vi "Calculate_10Minutes_Averages.vi"(0 "Current time":dbl) -> ()   [LabVIEW 2013]
uses:
  <vilib>/Analysis/baseanly.llb/Mean (DBL).vi
  Globals/Weather_Queues.vi
  <vilib>/Analysis/NI_AALBase.lvlib
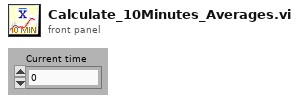
[diagram p1: front panel]
types:
  T1 = cluster{"Weather data (5s)":refnum<queue>, "Database queue":refnum<queue>, "Message queue":refnum<queue>, "Settings queue":refnum<queue>, "60 mins data queue":refnum<queue>, "48 hrs data queue":refnum<queue>}
  T2 = cluster{"Data out":dbl, "Data out":dbl, "Data out":dbl, "Data out":dbl, "Data out":dbl, "Data out":dbl, "Data out":dbl, "Data out":dbl, "Data out":dbl, "Data out":dbl, "Data out":dbl, "Data out":dbl, "Data out":dbl, "Data out":dbl, "seconds since 1Jan1904":dbl}[]
  T3 = cluster{"Data out":dbl, "Data out":dbl, "Data out":dbl, "Data out":dbl, "Data out":dbl, "Data out":dbl, "Data out":dbl, "Data out":dbl, "Data out":dbl, "Data out":dbl, "Data out":dbl, "Data out":dbl, "Data out":dbl, "Data out":dbl, "seconds since 1Jan1904":dbl}
  T4 = cluster{"mean":dbl, "mean":dbl, "mean":dbl, "mean":dbl, "mean":dbl, "mean":dbl, "mean":dbl, "mean":dbl, "mean":dbl, "mean":dbl, "mean":dbl, "mean":dbl, "mean":dbl, "mean":dbl, "mean":dbl}
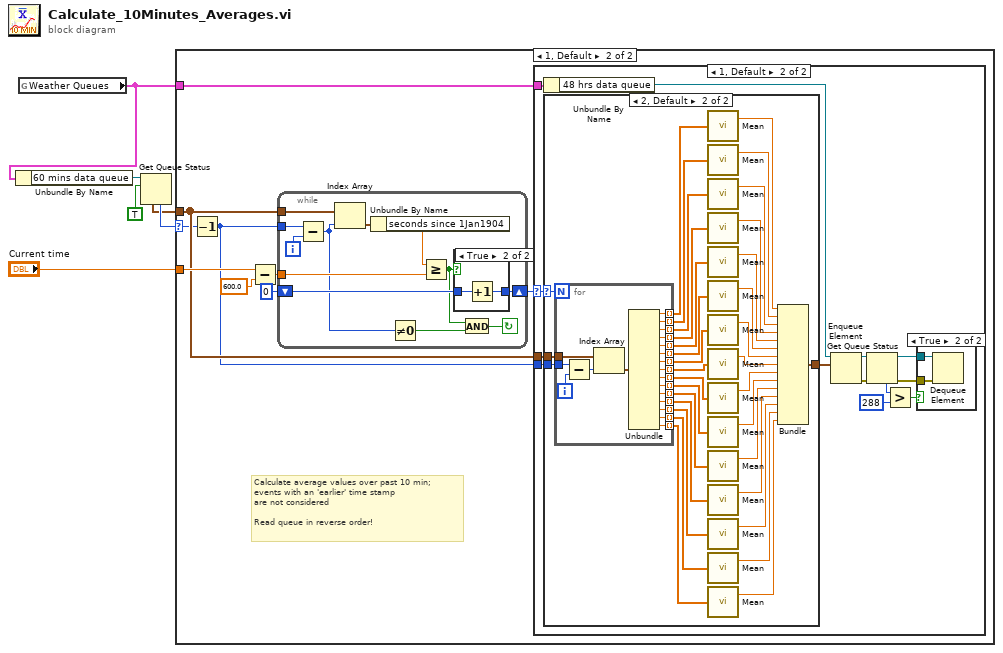
[diagram p0: block diagram]
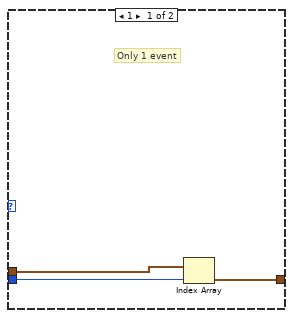
[diagram p6: hidden frame]
diagram:
  n1 = global read "Weather_Queues.vi" "Weather Queues"() -> (w1:T1)
  n2 = Unbundle By Name(w1) -> ("60 mins data queue"=w2:refnum<queue>)
  n3 = Get Queue Status(queue=w2, return elements? (F)=TRUE) -> (# elements in queue=w6:i32, elements=w5:T2)  [unwired: 1 in, 6 out]
  n4 = case shown="1, Default" w6 {
    selector: w6 -> [_ w9]
    tunnel: w5 -> [_ w10]
    tunnel: "Current time" -> [_ w11]
    tunnel: w1 -> [_ w7]
    frame 0 {
      # "No events"
    }
    frame 1, Default {
      # "Calculate average values over past 10 min;\nevents with an 'earlier' time stamp\nare not considered\n\nRead queue in reverse order!"
      n5 = Decrement(x=w9) -> (x-1=w8:i32)
      n6 = Subtract(x=w11, y=600.0) -> (x-y=w12:dbl)
      n7 = while {
        tunnel: w10 -> [w27]
        shift-right: [w26] -> w14
        shift-left: 0 -> [w25]
        tunnel: w12 -> [w22]
        tunnel: w8 -> [w21]
        i -> [w20]
        stop <- w18 continue-if-true
        n8 = Subtract(x=w21, y=w20) -> (x-y=w17:i32)
        n9 = Index Array(array=w27, index=w17) -> (element=w24:T3)
        n10 = Unbundle By Name(w24) -> ("seconds since 1Jan1904"=w23:dbl)
        n11 = Not Equal To 0?(x=w17) -> (x != 0?=w16:bool)
        n12 = Greater Or Equal?(x=w23, y=w22) -> (x >= y?=w19:bool)
        n13 = case shown="True" w19 {
          tunnel: w25 -> [w28 w29]
          tunnel: [w28 w30] -> w26
          frame False {
          }
          frame True {
            n14 = Increment(x=w29) -> (x+1=w30:i32)
          }
        }
        n15 = And(x=w19, y=w16) -> (x .and. y?=w18:bool)
      }
      n16 = case shown="1, Default" w14 {
        selector: w14 -> [_ w35]
        tunnel: w10 -> [_ w34]
        tunnel: w8 -> [_ w33]
        tunnel: w7 -> [_ w32]
        frame 0 {
          # "No events with a time stamp\nwithin past 600 seconds"
        }
        frame 1, Default {
          n17 = Unbundle By Name(w32) -> ("48 hrs data queue"=w31:refnum<queue>)
          n18 = case shown="2, Default" w35 {
            selector: w35 -> [_ w50]
            tunnel: [w48 w52] -> w36
            tunnel: w34 -> [w47 w51]
            tunnel: w33 -> [w46 w49]
            frame 1 {
              # "Only 1 event"
              n19 = Index Array(array=w47, index=w46) -> (element=w48:T3)
            }
            frame 2, Default {
              n20 = for {
                N: w50 -> [_]
                tunnel: [w102] -> w68 mode=indexing
                tunnel: [w101] -> w69 mode=indexing
                tunnel: [w100] -> w70 mode=indexing
                tunnel: [w99] -> w71 mode=indexing
                tunnel: [w98] -> w72 mode=indexing
                tunnel: [w97] -> w73 mode=indexing
                tunnel: [w96] -> w74 mode=indexing
                tunnel: [w95] -> w75 mode=indexing
                tunnel: [w94] -> w76 mode=indexing
                tunnel: [w93] -> w81 mode=indexing
                tunnel: [w92] -> w80 mode=indexing
                tunnel: [w89] -> w79 mode=indexing
                tunnel: [w91] -> w78 mode=indexing
                tunnel: [w90] -> w77 mode=indexing
                tunnel: [w88] -> w82 mode=indexing
                tunnel: w51 -> [w87]
                tunnel: w49 -> [w83]
                i -> [w85]
                n21 = Subtract(x=w83, y=w85) -> (x-y=w84:i32)
                n22 = Index Array(array=w87, index=w84) -> (element=w86:T3)
                n23 = Unbundle(w86) -> ("Data out"=w102:dbl, "Data out"=w101:dbl, "Data out"=w100:dbl, "Data out"=w99:dbl, "Data out"=w98:dbl, "Data out"=w97:dbl, "Data out"=w96:dbl, "Data out"=w95:dbl, "Data out"=w94:dbl, "Data out"=w93:dbl, "Data out"=w92:dbl, "Data out"=w89:dbl, "Data out"=w91:dbl, "Data out"=w90:dbl, "seconds since 1Jan1904"=w88:dbl)
              }
              n24 = call-poly <vilib>:"Mean.vi"("X"=w68) -> ("mean"=w54:dbl)  [unwired: 1 out]
              n25 = call-poly <vilib>:"Mean.vi"("X"=w69) -> ("mean"=w55:dbl)  [unwired: 1 out]
              n26 = call-poly <vilib>:"Mean.vi"("X"=w70) -> ("mean"=w56:dbl)  [unwired: 1 out]
              n27 = call-poly <vilib>:"Mean.vi"("X"=w71) -> ("mean"=w57:dbl)  [unwired: 1 out]
              n28 = call-poly <vilib>:"Mean.vi"("X"=w72) -> ("mean"=w58:dbl)  [unwired: 1 out]
              n29 = call-poly <vilib>:"Mean.vi"("X"=w73) -> ("mean"=w59:dbl)  [unwired: 1 out]
              n30 = call-poly <vilib>:"Mean.vi"("X"=w74) -> ("mean"=w60:dbl)  [unwired: 1 out]
              n31 = call-poly <vilib>:"Mean.vi"("X"=w75) -> ("mean"=w61:dbl)  [unwired: 1 out]
              n32 = call-poly <vilib>:"Mean.vi"("X"=w76) -> ("mean"=w62:dbl)  [unwired: 1 out]
              n33 = call-poly <vilib>:"Mean.vi"("X"=w81) -> ("mean"=w63:dbl)  [unwired: 1 out]
              n34 = call-poly <vilib>:"Mean.vi"("X"=w80) -> ("mean"=w64:dbl)  [unwired: 1 out]
              n35 = call-poly <vilib>:"Mean.vi"("X"=w79) -> ("mean"=w65:dbl)  [unwired: 1 out]
              n36 = call-poly <vilib>:"Mean.vi"("X"=w78) -> ("mean"=w66:dbl)  [unwired: 1 out]
              n37 = call-poly <vilib>:"Mean.vi"("X"=w77) -> ("mean"=w67:dbl)  [unwired: 1 out]
              n38 = call-poly <vilib>:"Mean.vi"("X"=w82) -> ("mean"=w53:dbl)  [unwired: 1 out]
              n39 = Bundle("mean"=w54, "mean"=w55, "mean"=w56, "mean"=w57, "mean"=w58, "mean"=w59, "mean"=w60, "mean"=w61, "mean"=w62, "mean"=w63, "mean"=w64, "mean"=w65, "mean"=w66, "mean"=w67, "mean"=w53) -> (w52:T4)  [unwired: 1 in]
            }
          }
          n40 = Enqueue Element(queue=w31, element=w36) -> (queue out=w43:refnum<queue>, error out=w42:errorcluster)  [unwired: 2 in, 1 out]
          n41 = Get Queue Status(queue=w43, error in (no error)=w42) -> (queue out=w39:refnum<queue>, error out=w38:errorcluster, # elements in queue=w40:i32)  [unwired: 1 in, 5 out]
          n42 = Greater?(x=w40, y=288) -> (0:w37:bool)
          n43 = case shown="True" w37 {
            tunnel: w38 -> [_ w44]
            tunnel: w39 -> [_ w45]
            frame False {
            }
            frame True {
              n44 = Dequeue Element(queue=w45, error in (no error)=w44) -> ()  [unwired: 1 in, 4 out]
            }
          }
        }
      }
    }
  }
